vi "TTRM Configure Thermistor Settings.vi"(0 "DAQmx Task In":refnum<k21>, 5 "Range and Terminal Settings":T1={"Global Settings"={"Min Temp (degC)"=0.0, "Max Temp (degC)"=100.0, "Vex Value (V)"=5.0, "R1 (Ohm)"=1000.0, "Terminal Configuration"=10083, "Thermistor Parameters"={"Type"=enum."Beta", "ABC Parameters"={"A"=0.001295361, "B"=0.0002343159, "C"=1.018703e-07}, "Beta Parameters"={"Beta Value (K)"=0.001295361, "R0 (Ohm)"=0.0002343159}}}, "Specific Channel Settings"=[]} {"Specific Channel Settings"."Terminal Configuration" items=["RSE"=10083, "NRSE"=10078, "Differential"=10106]; "Specific Channel Settings"."Thermistor Parameters"."Beta Parameters"."R0 (Ohm)" format="%#.6p"; "Specific Channel Settings"."Thermistor Parameters"."Beta Parameters"."Beta Value (K)" format="%.2f"; "Specific Channel Settings"."Thermistor Parameters"."ABC Parameters"."C" format="%^.6e"; "Specific Channel Settings"."Thermistor Parameters"."ABC Parameters"."B" format="%^.6e"; "Specific Channel Settings"."Thermistor Parameters"."ABC Parameters"."A" format="%^.6e"; "Specific Channel Settings"."R1 (Ohm)" format="%#.2p"; "Specific Channel Settings"."Vex Value (V)" format="%#.2p"; "Specific Channel Settings"."Max Temp (degC)" format="%.2f"; "Specific Channel Settings"."Min Temp (degC)" format="%.2f"; "Global Settings"."Terminal Configuration" items=["RSE"=10083, "NRSE"=10078, "Differential"=10106]; "Global Settings"."Thermistor Parameters"."Beta Parameters"."R0 (Ohm)" format="%#.6p"; "Global Settings"."Thermistor Parameters"."Beta Parameters"."Beta Value (K)" format="%#.6p"; "Global Settings"."Thermistor Parameters"."ABC Parameters"."C" format="%^.6e"; "Global Settings"."Thermistor Parameters"."ABC Parameters"."B" format="%^.6e"; "Global Settings"."Thermistor Parameters"."ABC Parameters"."A" format="%^.6e"; "Global Settings"."R1 (Ohm)" format="%#.2p"; "Global Settings"."Vex Value (V)" format="%#.2p"; "Global Settings"."Max Temp (degC)" format="%#.2p"; "Global Settings"."Min Temp (degC)" format="%#.2p"}, 11 "error in (no error)":errorcluster) -> (4 "DAQmx Task Out":refnum<k21>, 15 "error out":errorcluster)   [LabVIEW 2021, in "DAQ_Temperature Thermistor Measurement.lvlib"]
doc: "Configures the <B>Global and Specific</B> channels settings to the equivalent channels in DAQmx Task"
uses:
  DAQ_Temperature Thermistor Measurement.lvlib
  <resource>/objmgr/daqmx.rc
  Typedefs/Specific Channel Settings.ctl
  Typedefs/Range and Terminal Settings.ctl
  Typedefs/ABC Parameters.ctl
  Typedefs/Beta Parameters.ctl
  Typedefs/Thermistor Parameters.ctl
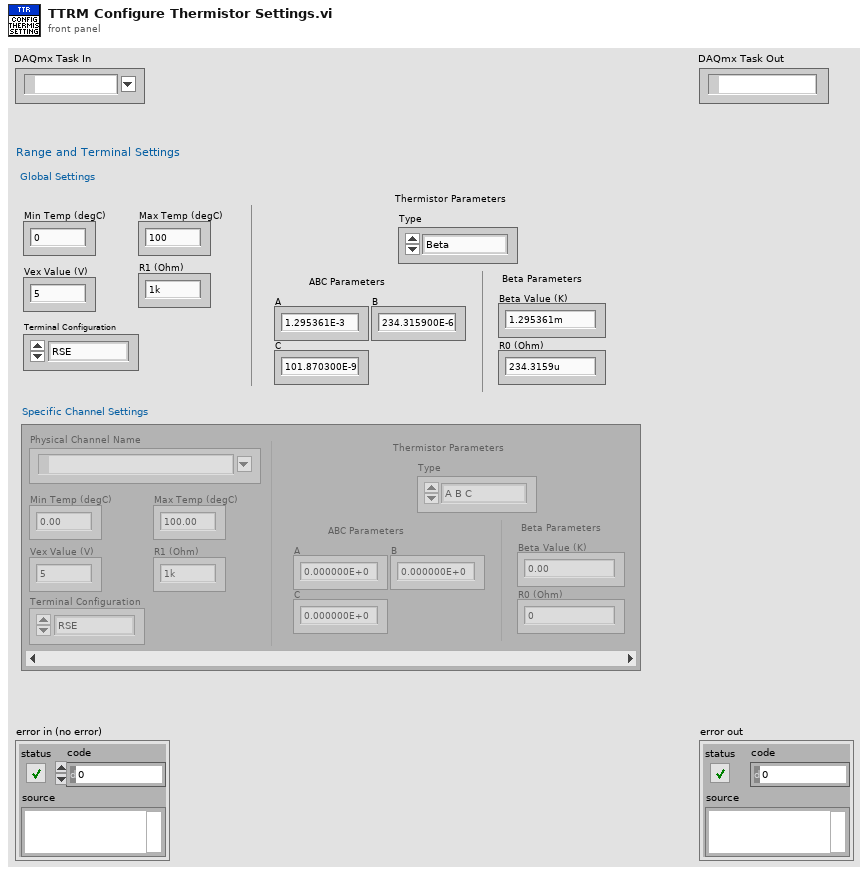
[diagram p1: front panel]
types:
  T1 = typedef "DAQ_Temperature Thermistor Measurement.lvlib/Range and Terminal Settings.ctl" = cluster{"Global Settings":cluster{"Min Temp (degC)":dbl, "Max Temp (degC)":dbl, "Vex Value (V)":dbl, "R1 (Ohm)":dbl, "Terminal Configuration":i32, "Thermistor Parameters":T2}, "Specific Channel Settings":T5[]}
  T2 = typedef "DAQ_Temperature Thermistor Measurement.lvlib/Thermistor Parameters.ctl" = cluster{"Type":enum16{"A B C", "Beta"}, "ABC Parameters":T3, "Beta Parameters":T4}
  T3 = typedef "DAQ_Temperature Thermistor Measurement.lvlib/ABC Parameters.ctl" = cluster{"A":dbl, "B":dbl, "C":dbl}
  T4 = typedef "DAQ_Temperature Thermistor Measurement.lvlib/Beta Parameters.ctl" = cluster{"Beta Value (K)":dbl, "R0 (Ohm)":dbl}
  T5 = typedef "DAQ_Temperature Thermistor Measurement.lvlib/Specific Channel Settings.ctl" = cluster{"Physical Channel Name":tag, "Min Temp (degC)":dbl, "Max Temp (degC)":dbl, "Vex Value (V) ":dbl, "R1 (Ohm)":dbl, "Terminal Configuration":i32, "Thermistor Parameters":T2}
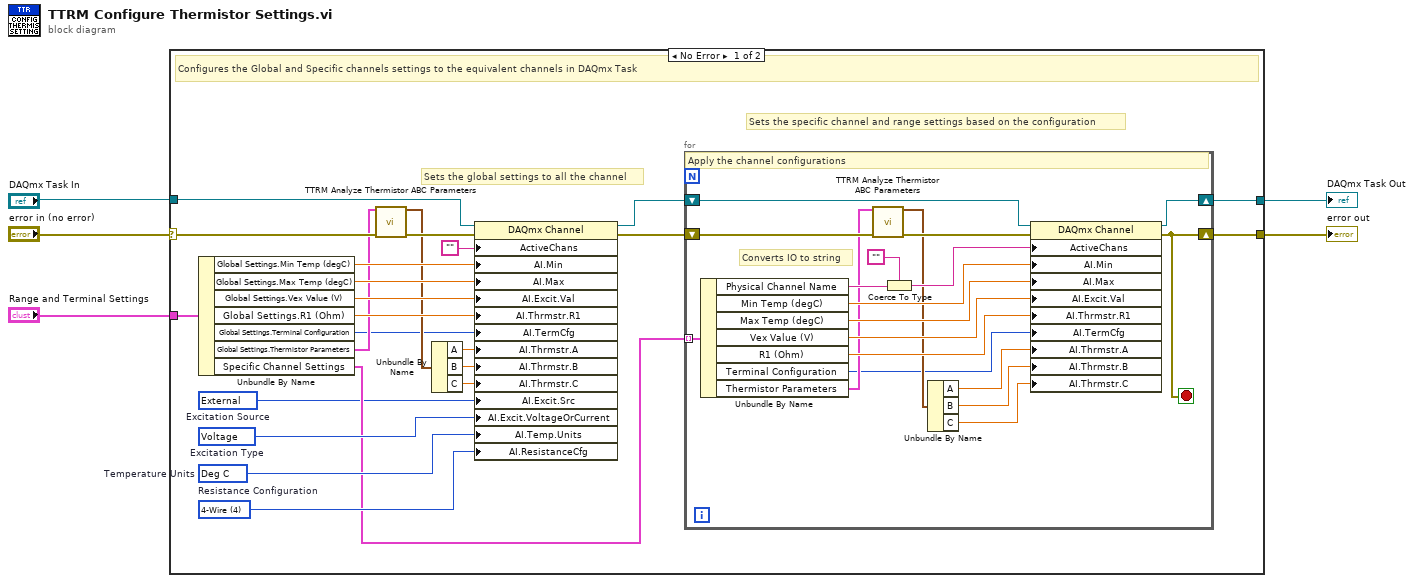
[diagram p0: block diagram]
diagram:
  n1 = case shown="No Error" "error in (no error)" {
    selector: "error in (no error)" -> [w17 w50]
    tunnel: "DAQmx Task In" -> [w26 w49]
    tunnel: "Range and Terminal Settings" -> [w24 _]
    tunnel: [w23 w49] -> w3
    tunnel: [w22 w50] -> w2
    frame No Error {
      w11 = 4 items=["2-Wire"=2, "3-Wire"=3, "4-Wire"=4]  # Resistance Configuration
      w18 = 10143 items=["Deg C"=10143, "Deg F"=10144, "Kelvins"=10325, "Deg R"=10145, "From Custom Scale"=10065]  # Temperature Units
      w19 = 10322 items=["Voltage"=10322, "Current"=10134]  # Excitation Type
      w6 = 10167 items=["Internal"=10200, "External"=10167, "None"=10230]  # Excitation Source
      # "Sets the specific channel and range settings based on the configuration"
      # "Sets the global settings to all the channel"
      # "Configures the Global and Specific channels settings to the equivalent channels in DAQmx Task"
      n2 = Unbundle By Name(w24) -> ("Global Settings.Min Temp (degC)"=w21:dbl, "Global Settings.Max Temp (degC)"=w29:dbl, "Global Settings.Vex Value (V)"=w20:dbl, "Global Settings.R1 (Ohm)"=w15:dbl, "Global Settings.Terminal Configuration"=w7:i32, "Global Settings.Thermistor Parameters"=w9:T2, "Specific Channel Settings"=w10:T5[])
      n3 = call "TTRM Analyze Thermistor ABC Parameters.vi"("Thermistor Parameters"=w9, "error in (no error)"=w17) -> ("ABC Parameters"=w14:T3, "error out"=w16:errorcluster)  [unwired: 12 in]
      n4 = Unbundle By Name(w14) -> ("A"=w8:dbl, "B"=w13:dbl, "C"=w12:dbl)
      n5 = property class="DAQmx Channel"(reference=w26, error in=w16, "ActiveChans"="", "AI.Min"=w21, "AI.Max"=w29, "AI.Excit.Val"=w20, "AI.Thrmstr.R1"=w15, "AI.TermCfg"=w7, "AI.Thrmstr.A"=w8, "AI.Thrmstr.B"=w13, "AI.Thrmstr.C"=w12, "AI.Excit.Src"=w6, "AI.Excit.VoltageOrCurrent"=w19, "AI.Temp.Units"=w18, "AI.ResistanceCfg"=w11) -> (reference out=w27:refnum<k21>, error out=w25:errorcluster)
      n6 = for {
        shift-right: [w47] -> w23
        shift-left: w27 -> [w48]
        shift-right: [w40] -> w22
        shift-left: w25 -> [w37]
        tunnel: w10 -> [w46] mode=indexing
        stop <- w40 stop-if-true
        # "Converts IO to string"
        # "Apply the channel configurations"
        n7 = Unbundle By Name(w46) -> ("Physical Channel Name"=w42:tag, "Min Temp (degC)"=w45:dbl, "Max Temp (degC)"=w44:dbl, "Vex Value (V)"=w39:dbl, "R1 (Ohm)"=w38:dbl, "Terminal Configuration"=w30:i32, "Thermistor Parameters"=w36:T2)
        n8 = call "TTRM Analyze Thermistor ABC Parameters.vi"("Thermistor Parameters"=w36, "error in (no error)"=w37) -> ("ABC Parameters"=w34:T3, "error out"=w35:errorcluster)  [unwired: 12 in]
        n9 = Coerce To Type(0:w42, 1:"") -> (2:w41:string)
        n10 = Unbundle By Name(w34) -> ("A"=w33:dbl, "B"=w32:dbl, "C"=w31:dbl)
        n11 = property class="DAQmx Channel"(reference=w48, error in=w35, "ActiveChans"=w41, "AI.Min"=w45, "AI.Max"=w44, "AI.Excit.Val"=w39, "AI.Thrmstr.R1"=w38, "AI.TermCfg"=w30, "AI.Thrmstr.A"=w33, "AI.Thrmstr.B"=w32, "AI.Thrmstr.C"=w31) -> (reference out=w47:refnum<k21>, error out=w40:errorcluster)
      }
    }
    frame Error {
    }
  }
  "DAQmx Task Out" <- w3
  "error out" <- w2
